vi "event read.vi"() -> ()   [LabVIEW 2020]
uses:
  MIDIllan/midi status byte.ctl
  MIDIllan/midi note name.ctl
  midi in/midi in.lvclass
  MIDIllan/MIDIllan.lvlib
panel:
  out "note name":T1
  out "MIDI Status Byte":T2
  out "MIDI Device Name":string
  out "raw_status":i32
  out "velocity_or_value":i32
  out "channel":i32
  out "message type":i32
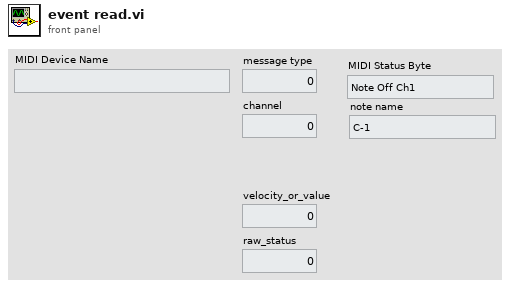
[diagram p1: front panel]
types:
  T1 = typedef "MIDIllan.lvlib/midi note name.ctl" = enum8{"C-1", "C#-1", "D-1", "D#-1", "E-1", "F-1", "F#-1", "G-1", "G#-1", "A-1", "A#-1", "B-1", "C0", "C#0", "D0", "D#0", "E0", "F0", "F#0", "G0", "G#0", "A0", "A#0", "B0", "C1", "C#1", "D1", "D#1", "E1", "F1", "F#1", "G1", "G#1", "A1", "A#1", "B1", "C2", "C#2", "D2", "D#2", "E2", "F2", "F#2", "G2", "G#2", "A2", "A#2", "B2", "C3", "C#3", "D3", "D#3", "E3", "F3", "F#3", "G3", "G#3", "A3", "A#3", "B3", "C4", "C#4", "D4", "D#4", "E4", "F4", "F#4", "G4", "G#4", "A4", "A#4", "B4", "C5", "C#5", "D5", "D#5", "E5", "F5", "F#5", "G5", "G#5", "A5", "A#5", "B5", "C6", "C#6", "D6", "D#6", "E6", "F6", "F#6", "G6", "G#6", "A6", "A#6", "B6", "C7", "C#7", "D7", "D#7", "E7", "F7", "F#7", "G7", "G#7", "A7", "A#7", "B7", "C8", "C#8", "D8", "D#8", "E8", "F8", "F#8", "G8", "G#8", "A8", "A#8", "B8", "C9", "C#9", "D9", "D#9", "E9", "F9", "F#9", "G9", "G#9", "A9", "A#9", "B9", "C10", "C#10", "D10", "D#10", "E10", "F10", "F#10", "G10"}
  T2 = typedef "MIDIllan.lvlib/midi status byte.ctl" = enum8{"Note Off Ch1", "Note Off Ch2", "Note Off Ch3", "Note Off Ch4", "Note Off Ch5", "Note Off Ch6", "Note Off Ch7", "Note Off Ch8", "Note Off Ch9", "Note Off Ch10", "Note Off Ch11", "Note Off Ch12", "Note Off Ch13", "Note Off Ch14", "Note Off Ch15", "Note Off Ch16", "Note On Ch1", "Note On Ch2", "Note On Ch3", "Note On Ch4", "Note On Ch5", "Note On Ch6", "Note On Ch7", "Note On Ch8", "Note On Ch9", "Note On Ch10", "Note On Ch11", "Note On Ch12", "Note On Ch13", "Note On Ch14", "Note On Ch15", "Note On Ch16", "Poly Aftertouch Ch1", "Poly Aftertouch Ch2", "Poly Aftertouch Ch3", "Poly Aftertouch Ch4", "Poly Aftertouch Ch5", "Poly Aftertouch Ch6", "Poly Aftertouch Ch7", "Poly Aftertouch Ch8", "Poly Aftertouch Ch9", "Poly Aftertouch Ch10", "Poly Aftertouch Ch11", "Poly Aftertouch Ch12", "Poly Aftertouch Ch13", "Poly Aftertouch Ch14", "Poly Aftertouch Ch15", "Poly Aftertouch Ch16", "Control Change Ch1", "Control Change Ch2", "Control Change Ch3", "Control Change Ch4", "Control Change Ch5", "Control Change Ch6", "Control Change Ch7", "Control Change Ch8", "Control Change Ch9", "Control Change Ch10", "Control Change Ch11", "Control Change Ch12", "Control Change Ch13", "Control Change Ch14", "Control Change Ch15", "Control Change Ch16", "Program Change Ch1", "Program Change Ch2", "Program Change Ch3", "Program Change Ch4", "Program Change Ch5", "Program Change Ch6", "Program Change Ch7", "Program Change Ch8", "Program Change Ch9", "Program Change Ch10", "Program Change Ch11", "Program Change Ch12", "Program Change Ch13", "Program Change Ch14", "Program Change Ch15", "Program Change Ch16", "Channel Aftertouch Ch1", "Channel Aftertouch Ch2", "Channel Aftertouch Ch3", "Channel Aftertouch Ch4", "Channel Aftertouch Ch5", "Channel Aftertouch Ch6", "Channel Aftertouch Ch7", "Channel Aftertouch Ch8", "Channel Aftertouch Ch9", "Channel Aftertouch Ch10", "Channel Aftertouch Ch11", "Channel Aftertouch Ch12", "Channel Aftertouch Ch13", "Channel Aftertouch Ch14", "Channel Aftertouch Ch15", "Channel Aftertouch Ch16", "Pitch Bend Ch1", "Pitch Bend Ch2", "Pitch Bend Ch3", "Pitch Bend Ch4", "Pitch Bend Ch5", "Pitch Bend Ch6", "Pitch Bend Ch7", "Pitch Bend Ch8", "Pitch Bend Ch9", "Pitch Bend Ch10", "Pitch Bend Ch11", "Pitch Bend Ch12", "Pitch Bend Ch13", "Pitch Bend Ch14", "Pitch Bend Ch15", "Pitch Bend Ch16", "System Exclusive Start", "MIDI Time Code Quarter Frame", "Song Position Pointer", "Song Select", "System Common Undefined F4", "System Common Undefined F5", "Tune Request", "System Exclusive End", "Timing Clock", "System Real-time Undefined F9", "Start", "Continue", "Stop", "System Real-time Undefined FD", "Active Sensing", "System Reset"}
  T3 = cluster{"message type":i32, "channel":i32, "note_or_controller":i32, "velocity_or_value":i32, "raw_status":i32}
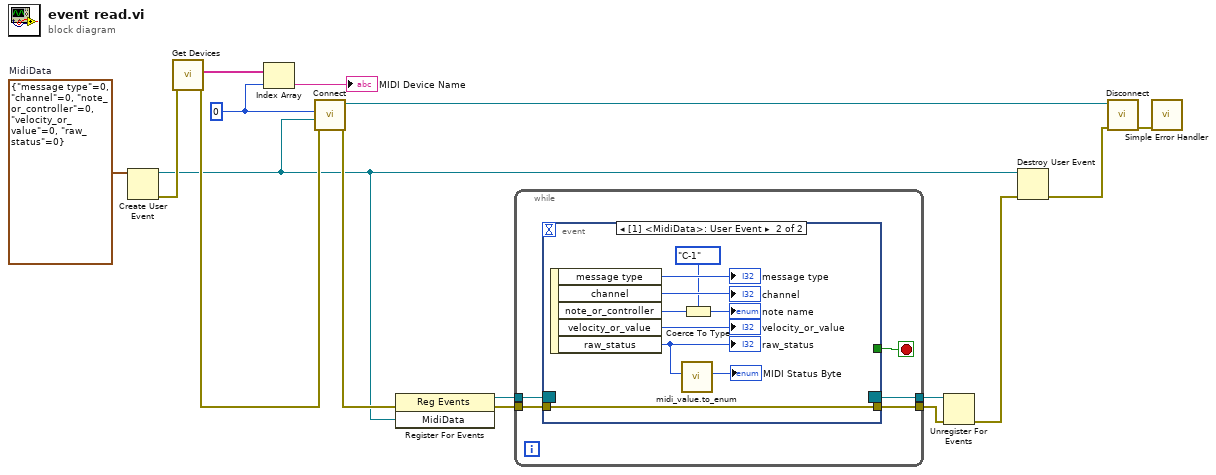
[diagram p0: block diagram]
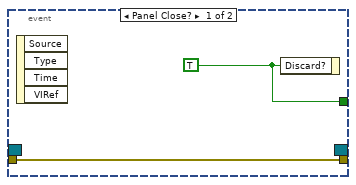
[diagram p2: hidden frame]
diagram:
  w8 = 0 ("index")
  w14 = T3 {"message type"=0, "channel"=0, "note_or_controller"=0, "velocity_or_value"=0, "raw_status"=0}  # MidiData
  n1 = Create User Event(user event datatype=w14) -> (user event=w1:refnum<user-event>, error out=w5:errorcluster)  [unwired: 1 in]
  n2 = call "Get Devices.vi"("error in (no error)"=w5) -> ("error out"=w6:errorcluster, "Device Names"=w9:string[])  [unwired: 9 in]
  n3 = Index Array(array=w9, index=w8) -> (element=→"MIDI Device Name":string)
  n4 = call "Connect.vi"("error in (no error)"=w6, "MIDI Data"=w1, "Device Index"=w8) -> ("error out"=w10:errorcluster, "midi in"=w11:refnum<class "midi in.lvclass">)  [unwired: 7 in]
  n5 = register-events(error in=w10, w1) -> (reference out=w13:refnum<event-registration>, error out=w12:errorcluster)  [unwired: 1 in]
  n6 = while {
    tunnel: w13 -> [w20]
    tunnel: [w19] -> w16
    tunnel: w12 -> [w18]
    tunnel: [w17] -> w2
    stop <- w21 stop-if-true
    n7 = event shown="[1] <MidiData>: User Event" {
      selector: w20 -> [_ _]
      dyn-events: [_ _] -> w19
      timeout: _ -> [_ _]
      tunnel: [w23 _] -> w21
      tunnel: w18 -> [w22 w29]
      tunnel: [w22 w29] -> w17
      event Panel Close? {
        w23 = TRUE ("Discard?")
        n8 = event-data() -> ()  [unwired: 1 in, 4 out]
        n9 = event-data("Discard?"=w23) -> ()  [unwired: 1 in, 1 out]
      }
      event User Event {
        n10 = event-data() -> ("message type"=→"message type":i32, "channel"=→"channel":i32, "note_or_controller"=w26:i32, "velocity_or_value"=→"velocity_or_value":i32, "raw_status"=w28:i32)  [unwired: 1 in]
        "raw_status" <- w28
        n11 = call "midi_value.to_enum.vi"("midi value"=w28) -> ("MIDI Status Byte"=→"MIDI Status Byte":T2)  [unwired: 10 in]
        n12 = Coerce To Type(0:w26, 1:midi_note_name."C-1" ("MIDI Status Byte")) -> (2:→"note name":T1)
      }
    }
  }
  n13 = Unregister For Events(event registration refnum=w16, error in=w2) -> (error out=w15:errorcluster)
  n14 = Destroy User Event(user event=w1, error in=w15) -> (error out=w4:errorcluster)
  n15 = call "Disconnect.vi"("error in (no error)"=w4, "midi in in"=w11) -> ("error out"=w3:errorcluster)  [unwired: 9 in]
  n16 = call <vilib>:"Simple Error Handler.vi"("error in (no error)"=w3) -> ()  [unwired: 4 in, 5 out]
